vi "8 Bits Read.vi"(6 "E?E1:E2 (E1)":bool=TRUE, 9 "RS":bool, 11 "device connection map":T1={"RS"="RS", "R/W"="RW", "E1"="E1", "E2"="E1", "DB0"="DB0", "DB1"="DB1", "DB2"="DB2", "DB3"="DB3", "DB4"="DB4", "DB5"="DB5", "DB6"="DB6", "DB7"="DB7"}) -> (1 "value":u8)   [LabVIEW 2017, in "HD44780 FPGA.lvlib"]
uses:
  HD44780 FPGA.lvlib
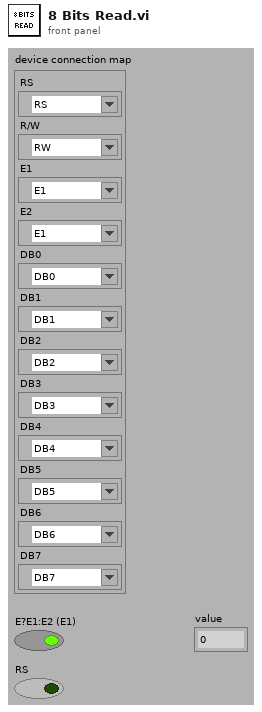
[diagram p1: front panel]
types:
  T1 = cluster{"RS":refnum<k21>, "R/W":refnum<k21>, "E1":refnum<k21>, "E2":refnum<k21>, "DB0":refnum<k21>, "DB1":refnum<k21>, "DB2":refnum<k21>, "DB3":refnum<k21>, "DB4":refnum<k21>, "DB5":refnum<k21>, "DB6":refnum<k21>, "DB7":refnum<k21>}
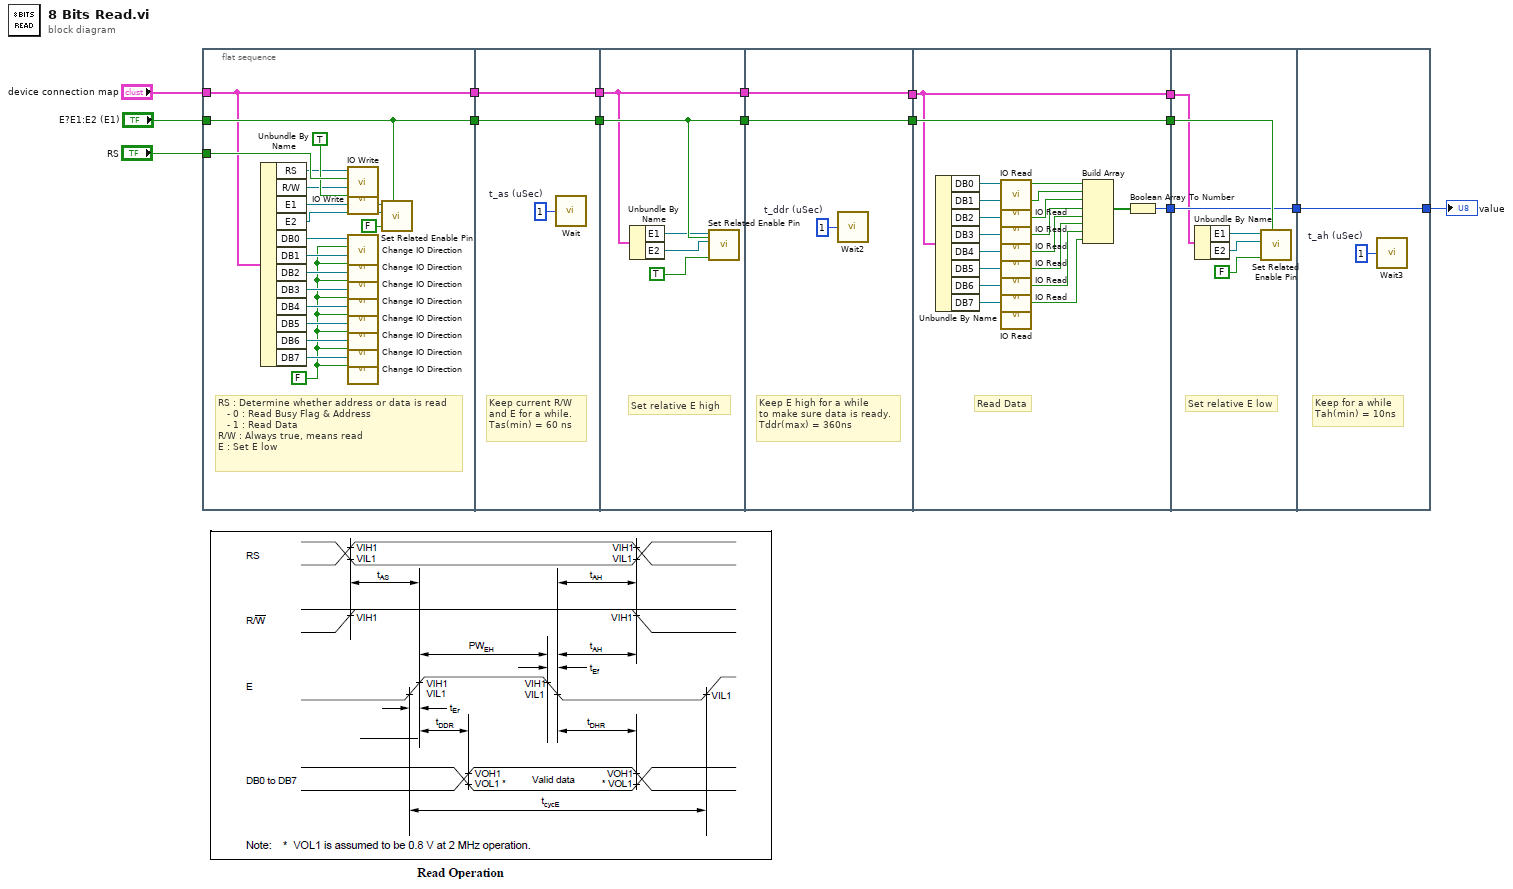
[diagram p0: block diagram]
diagram:
  n1 = flat-sequence {
    tunnel: [w30] -> w2
    tunnel: "RS" -> [w34]
    tunnel: "E?E1:E2 (E1)" -> [w30]
    tunnel: "device connection map" -> [w17]
    tunnel: [w17] -> w1
    tunnel: w2 -> [w36]
    tunnel: [w36] -> w13
    tunnel: [w35] -> w5
    tunnel: w1 -> [w35]
    tunnel: w13 -> [w41]
    tunnel: [w41] -> w12
    tunnel: [w38] -> w6
    tunnel: w5 -> [w38]
    tunnel: w12 -> [w44]
    tunnel: [w44] -> w11
    tunnel: [w43] -> w7
    tunnel: w6 -> [w43]
    tunnel: [w65] -> w10
    tunnel: w11 -> [w55]
    tunnel: [w55] -> w9
    tunnel: w7 -> [w46]
    tunnel: [w46] -> w4
    tunnel: w10 -> [w69]
    tunnel: [w69] -> w8
    tunnel: w9 -> [w71]
    tunnel: w4 -> [w68]
    tunnel: [w72] -> w15
    tunnel: w8 -> [w72]
    frame #0 {
      w18 = FALSE ("T? write:read")
      # "RS : Determine whether address or data is read\n   - 0 : Read Busy Flag & Address  \n   - 1 : Read Data\nR/W : Always true, means read\nE : Set E low"
      n2 = Unbundle By Name(w17) -> ("RS"=w32:refnum<k21>, "R/W"=w31:refnum<k21>, "E1"=w29:refnum<k21>, "E2"=w28:refnum<k21>, "DB0"=w26:refnum<k21>, "DB1"=w25:refnum<k21>, "DB2"=w24:refnum<k21>, "DB3"=w23:refnum<k21>, "DB4"=w22:refnum<k21>, "DB5"=w21:refnum<k21>, "DB6"=w20:refnum<k21>, "DB7"=w19:refnum<k21>)
      n3 = call "IO Write.vi"("data"=w34, "I/O"=w32) -> ()  [unwired: 10 in]
      n4 = call "IO Write.vi"("data"=TRUE ("Data"), "I/O"=w31) -> ()  [unwired: 10 in]
      n5 = call "Change IO Direction.vi"("T? write:read"=w18, "I/O"=w26) -> ()  [unwired: 10 in]
      n6 = call "Change IO Direction.vi"("T? write:read"=w18, "I/O"=w25) -> ()  [unwired: 10 in]
      n7 = call "Change IO Direction.vi"("T? write:read"=w18, "I/O"=w24) -> ()  [unwired: 10 in]
      n8 = call "Change IO Direction.vi"("T? write:read"=w18, "I/O"=w23) -> ()  [unwired: 10 in]
      n9 = call "Change IO Direction.vi"("T? write:read"=w18, "I/O"=w22) -> ()  [unwired: 10 in]
      n10 = call "Change IO Direction.vi"("T? write:read"=w18, "I/O"=w21) -> ()  [unwired: 10 in]
      n11 = call "Change IO Direction.vi"("T? write:read"=w18, "I/O"=w20) -> ()  [unwired: 10 in]
      n12 = call "Change IO Direction.vi"("T? write:read"=w18, "I/O"=w19) -> ()  [unwired: 10 in]
      n13 = call "Set Related Enable Pin.vi"("E?E1:E2"=w30, "data"=FALSE, "E2"=w28, "E1"=w29) -> ()  [unwired: 8 in]
    }
    frame #1 {
      w37 = u8 1  # t_as (uSec)
      # "Keep current R/W \nand E for a while.  \nTas(min) = 60 ns"
      n14 = call "Wait"("Count(uSec)"=w37) -> ()  [unwired: 1 out]
    }
    frame #2 {
      # "Set relative E high"
      n15 = Unbundle By Name(w38) -> ("E1"=w40:refnum<k21>, "E2"=w39:refnum<k21>)
      n16 = call "Set Related Enable Pin.vi"("E?E1:E2"=w41, "data"=TRUE, "E2"=w39, "E1"=w40) -> ()  [unwired: 8 in]
    }
    frame #3 {
      w45 = u8 1  # t_ddr (uSec)
      # "Keep E high for a while\nto make sure data is ready.\nTddr(max) = 360ns"
      n17 = call "Wait2"("Count(uSec)"=w45) -> ()  [unwired: 1 out]
    }
    frame #4 {
      # "Read Data"
      n18 = Unbundle By Name(w46) -> ("DB0"=w47:refnum<k21>, "DB1"=w48:refnum<k21>, "DB2"=w49:refnum<k21>, "DB3"=w50:refnum<k21>, "DB4"=w51:refnum<k21>, "DB5"=w52:refnum<k21>, "DB6"=w53:refnum<k21>, "DB7"=w54:refnum<k21>)
      n19 = call "IO Read.vi"("I/O"=w47) -> ("data"=w64:bool)  [unwired: 10 in]
      n20 = call "IO Read.vi"("I/O"=w48) -> ("data"=w63:bool)  [unwired: 10 in]
      n21 = call "IO Read.vi"("I/O"=w49) -> ("data"=w62:bool)  [unwired: 10 in]
      n22 = call "IO Read.vi"("I/O"=w50) -> ("data"=w61:bool)  [unwired: 10 in]
      n23 = call "IO Read.vi"("I/O"=w51) -> ("data"=w60:bool)  [unwired: 10 in]
      n24 = call "IO Read.vi"("I/O"=w52) -> ("data"=w59:bool)  [unwired: 10 in]
      n25 = call "IO Read.vi"("I/O"=w53) -> ("data"=w58:bool)  [unwired: 10 in]
      n26 = call "IO Read.vi"("I/O"=w54) -> ("data"=w57:bool)  [unwired: 10 in]
      n27 = Build Array(w64, w63, w62, w61, w60, w59, w58, w57) -> (w56:bool[])
      n28 = Boolean Array To Number(Boolean array=w56) -> (number=w65:u8)
    }
    frame #5 {
      # "Set relative E low"
      n29 = Unbundle By Name(w68) -> ("E1"=w67:refnum<k21>, "E2"=w66:refnum<k21>)
      n30 = call "Set Related Enable Pin.vi"("E?E1:E2"=w71, "data"=FALSE, "E2"=w66, "E1"=w67) -> ()  [unwired: 8 in]
    }
    frame #6 {
      w73 = u8 1  # t_ah (uSec)
      # "Keep for a while\nTah(min) = 10ns"
      n31 = call "Wait3"("Count(uSec)"=w73) -> ()  [unwired: 1 out]
    }
  }
  "value" <- w15
